vi "List Compatible Ctls.vi"(11 "Visible UIP In":refnum<class "VisibleUIP.lvclass">) -> (2 "Compatible Ctl Classes":string[](array[string]), 3 "Visible UIP Out":refnum<class "VisibleUIP.lvclass">)   [LabVIEW 2015, in "VisibleUIP.lvclass"]
doc: "Overwrite this method in your child UIPs to provide a custom list of vi server control classes compatible with that UIP."
uses:
  VisibleUIP.lvclass
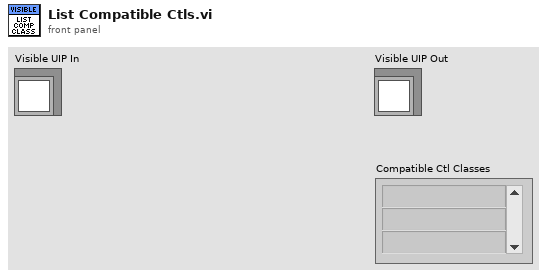
[diagram p1: front panel]
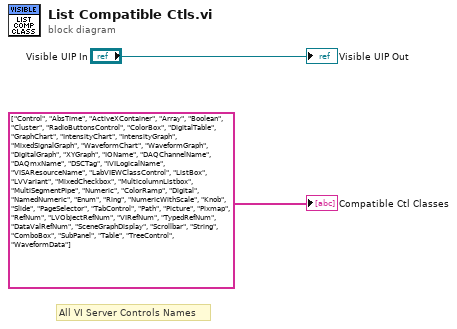
[diagram p0: block diagram]
diagram:
  # "All VI Server Controls Names"
  "Compatible Ctl Classes" <- string[] ["Control", "AbsTime", "ActiveXContainer", "Array", "Boolean", "Cluster", "RadioButtonsControl", "ColorBox", "DigitalTable", "GraphChart", "IntensityChart", "IntensityGraph", "MixedSignalGraph", "WaveformChart", "WaveformGraph", "DigitalGraph", "XYGraph", "IOName", "DAQChannelName", "DAQmxName", "DSCTag", "IVILogicalName", "VISAResourceName", "LabVIEWClassControl", "ListBox", "LVVariant", "MixedCheckbox", "MulticolumnListbox", "MultiSegmentPipe", "Numeric", "ColorRamp", "Digital", "NamedNumeric", "Enum", "Ring", "NumericWithScale", "Knob", "Slide", "PageSelector", "TabControl", "Path", "Picture", "Pixmap", "RefNum", "LVObjectRefNum", "VIRefNum", "TypedRefNum", "DataValRefNum", "SceneGraphDisplay", "Scrollbar", "String", "ComboBox", "SubPanel", "Table", "TreeControl", "WaveformData"]
  "Visible UIP Out" <- "Visible UIP In"
